vi "DSF.Engine.Builder.Send Response.vi"(8 "error in (no error)":errorcluster, 10 "response":T1, 11 "Builder in":refnum<class "DSF.Engine.Builder.lvclass">) -> (0 "error out":errorcluster, 3 "Builder out":refnum<class "DSF.Engine.Builder.lvclass">)   [LabVIEW 2017, in "DSF.Engine.lvlib" / "DSF.Engine.Builder.lvclass"]
uses:
  DSF.Engine.Builder.lvclass
  Interface/DSF.Engine.Interface.Builder.Response Data.ctl
  Interface/DSF.Engine.Interface.Builder.Response.ctl
  DSF.Engine.Builder.lvclass/DSF.Engine.Builder.ctl
  Interface/DSF.Engine.Interface.Builder.Write.Response.vi
  Interface/DSF.Engine.Interface.Builder.lvclass
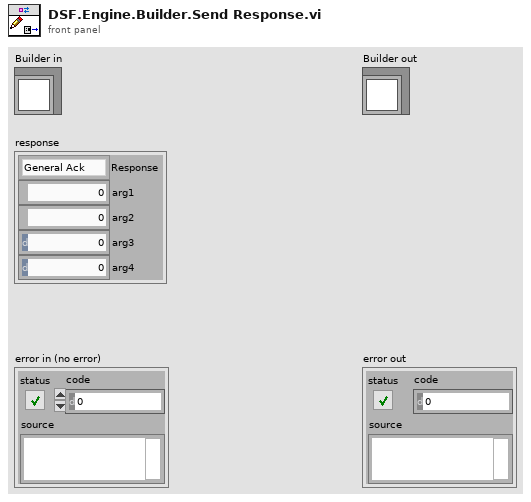
[diagram p1: front panel]
types:
  T1 = typedef "DSF.Engine.lvlib/DSF.Engine.Interface.Builder.lvclass/DSF.Engine.Interface.Builder.Response Data.ctl" = cluster{"Response":T2, "arg1":i32, "arg2":i32, "arg3":i32, "arg4":i32}
  T2 = typedef "DSF.Engine.lvlib/DSF.Engine.Interface.Builder.lvclass/DSF.Engine.Interface.Builder.Response.ctl" = enum8{"General Ack", "Initialize Complete", "Build Complete", "Parse Complete", "Shutdown Ack"}
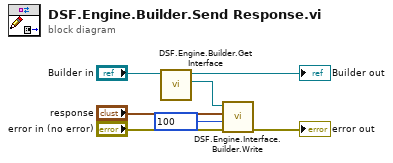
[diagram p0: block diagram]
diagram:
  n1 = call "DSF.Engine.Builder.Get Interface.vi"("Builder in"="Builder in") -> ("Builder Interface"=w5:refnum<class "DSF.Engine.Interface.Builder.lvclass">, "Builder out"=→"Builder out":refnum<class "DSF.Engine.Builder.lvclass">)  [unwired: 9 in]
  n2 = call-poly "DSF.Engine.Interface.Builder.Write.vi"("error in (no error)"="error in (no error)", "timeout in ms (0)"=100, "response"="response", "Builder Interface in"=w5) -> ("error out"=→"error out":errorcluster)  [unwired: 5 in, 2 out]
